vi "SpinnyStartMove.vi"(0 "Arduino Resource":T1={"VISA resource"="", "Board Type"=enum."Uno", "Connection Type"=enum."USB / Serial", "Bytes Per Packet (15)"=15}, 5 "Degrees To Move":sgl, 7 "Steps Per Degree":u32=50, 9 "Direction":i8=1, 11 "error in":errorcluster, 12 "Stepper#":u8=1, 13 "Max Speed (steps/s)":u16=450, 14 "Acceleration (steps/s/s)":u16=100) -> (4 "Arduino Resource Out":T1={"VISA resource"="", "Board Type"=enum."Uno", "Connection Type"=enum."USB / Serial", "Bytes Per Packet (15)"=15}, 15 "error out":errorcluster)   [LabVIEW 2014]
doc: "Move the rotator"
uses:
  <vilib>/LabVIEW Interface for Arduino/Type Defs/Arduino Resource.ctl
  <vilib>/LabVIEW Interface for Arduino/Type Defs/Board Type.ctl
  <vilib>/LabVIEW Interface for Arduino/LabVIEW Interface for Arduino.lvlib
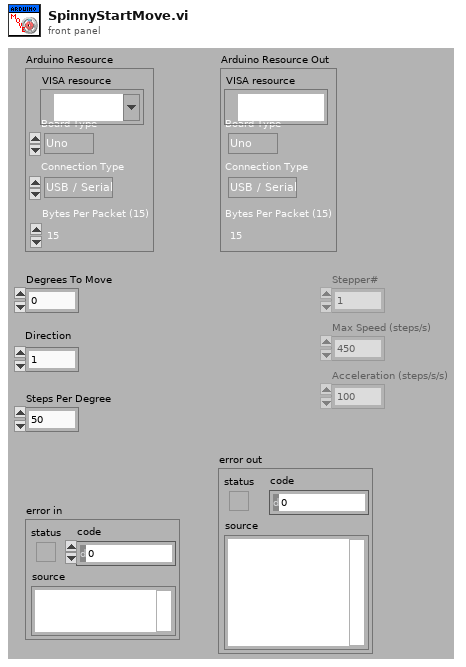
[diagram p1: front panel]
types:
  T1 = typedef "LabVIEW Interface for Arduino.lvlib/Arduino Resource.ctl" = cluster{"VISA resource":refnum<visa-resource-name>, "Board Type":T2, "Connection Type":enum8{"USB / Serial"}, "Bytes Per Packet (15)":u8}
  T2 = typedef "LabVIEW Interface for Arduino.lvlib/Board Type.ctl" = enum16{"Uno", "Dimuelanove w/Atmega 328", "Mega 2560"}
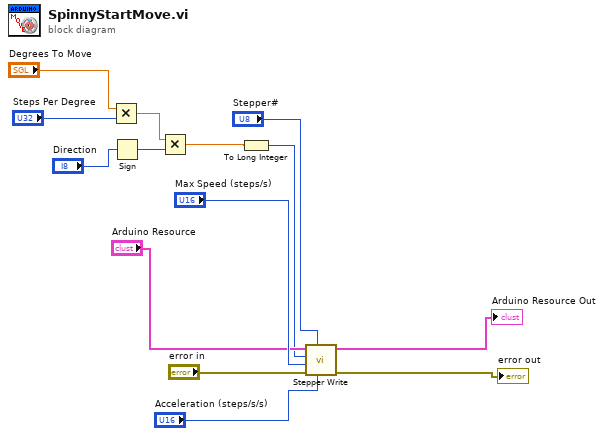
[diagram p0: block diagram]
diagram:
  n1 = Multiply(x="Degrees To Move", y="Steps Per Degree") -> (x*y=w3:sgl)
  n2 = Sign(1:"Direction") -> (0:w10:i8)
  n3 = Multiply(x=w3, y=w10) -> (x*y=w2:sgl)
  n4 = To Long Integer(number=w2) -> (32bit integer=w1:i32)
  n5 = call <vilib>:"Stepper Write.vi"("Set Acceleration (0 to disable)"="Acceleration (steps/s/s)", "Stepper #"="Stepper#", "error in"="error in", "Set Speed (Steps per Second)"="Max Speed (steps/s)", "# of Steps to Move"=w1, "Arduino Resource"="Arduino Resource") -> ("error out"=→"error out":errorcluster, "Arduino Resource Out"=→"Arduino Resource Out":T1)  [unwired: 4 in]
